vi "插入单条数据.vi"(8 "错误输入（无错误）":errorcluster, 10 "table输入":string(combo), 11 "插入数据":string[](array[string])) -> (0 "错误输出":errorcluster, 3 "远程数据":string[][](table))   [LabVIEW 2016]
uses:
  <vilib>/Utility/sysdir.llb/System Directory Type.ctl
  <vilib>/addons/database/Connection.llb/DB Tools Open Connec (String).vi
  <vilib>/addons/database/Connection.llb/Conn Execute.vi
  <vilib>/addons/database/Recordset.llb/Rec Destroy - Connection.vi
  <vilib>/addons/database/_DB Variant To Data/Database Variant To Data.xnode
  <vilib>/addons/database/NI_Database_API.lvlib
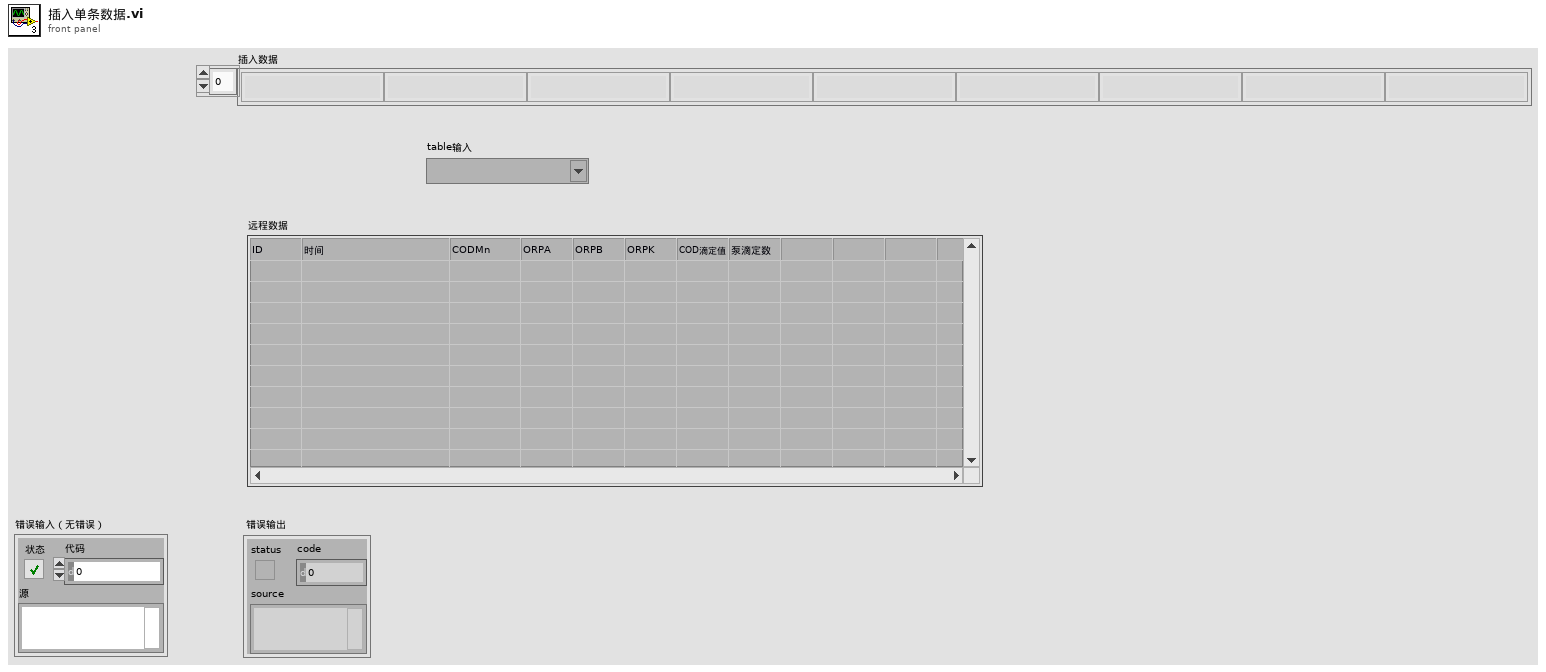
[diagram p1: front panel]
types:
  T1 = typedef "System Directory Type.ctl" = i32
  T2 = typedef "NI_Database_API.lvlib/Conn ObjectReference.ctl" = refnum<k1>
  T3 = typedef "NI_Database_API.lvlib/Rec ObjectReference.ctl" = refnum<k1>
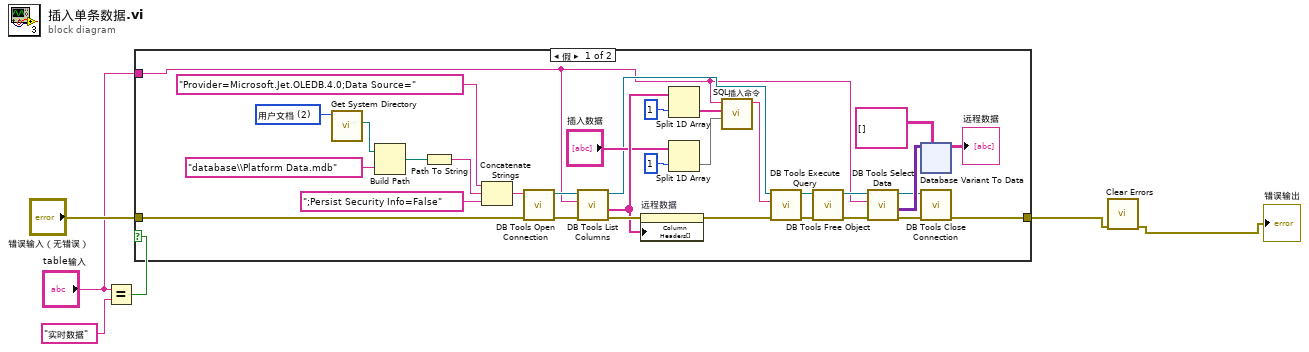
[diagram p0: block diagram]
diagram:
  n1 = Equal?(x="table输入", y="实时数据") -> (x = y?=w3:bool)
  n2 = case shown="假" w3 {
    tunnel: [w38 w83] -> w2
    tunnel: "错误输入（无错误）" -> [w20 w83]
    tunnel: "table输入" -> [w7 _]
    frame False {
      w21 = T1 2 items=["用户目录"=0, "用户桌面"=1, "用户文档"=2, "用户应用程序数据"=3, "用户设置"=4, "用户临时目录"=5, "公共文档"=6, "公共应用程序数据"=7, "公共设置"=8, "公共缓存"=13, "系统核心库"=9, "系统安装库"=10, "应用程序文件"=11, "启动盘根目录"=12] ("system directory type")
      n3 = call <vilib>:"Get System Directory.vi"("system directory type"=w21) -> ("system directory"=w23:path)  [unwired: 10 in]
      n4 = Build Path(base path=w23, name or relative path="database\\Platform Data.mdb" ("condition")) -> (appended path=w24:path)
      n5 = Path To String(path=w24) -> (string=w25:string)
      n6 = Concatenate Strings("Provider=Microsoft.Jet.OLEDB.4.0;Data Source=" ("condition"), w25, ";Persist Security Info=False" ("condition")) -> (w27:string)
      n7 = call-poly <vilib>:"DB Tools Open Connection.vi"("error in (no error)"=w20, "connection information"=w27) -> ("error out"=w36:errorcluster, "connection reference"=w35:T2)  [unwired: 6 in]
      n8 = call <vilib>:"DB Tools List Columns.vi"("error in (no error)"=w36, "table"=w7, "connection reference"=w35) -> ("error out"=w19:errorcluster, "columns"=w18:string[], "connection reference out"=w15:T2)  [unwired: 1 in, 1 out]
      n9 = property on="远程数据" class="Tbl (严格)"(error in=w19, "Column Headers[]"=w18) -> (error out=w14:errorcluster)  [unwired: 1 in, 1 out]
      n10 = Split 1D Array(array=w18, index=1 ("索引")) -> (second subarray=w9:string[])  [unwired: 1 out]
      n11 = Split 1D Array(array="插入数据", index=1 ("索引")) -> (second subarray=w8:string[])  [unwired: 1 out]
      n12 = call "SQL插入命令.vi"("插入数值"=w8, "段名"=w9, "table"=w7) -> ("SQL插入命令"=w16:string)  [unwired: 8 in]
      n13 = call-poly <vilib>:"DB Tools Execute Query.vi"("error in (no error)"=w14, "SQL query"=w16, "connection reference"=w15) -> ("error out"=w12:errorcluster, "recordset reference"=w13:T3)  [unwired: 5 in]
      n14 = call-poly <vilib>:"DB Tools Free Object.vi"("error in (no error)"=w12, "recordset reference"=w13) -> ("error out"=w10:errorcluster, "connection reference"=w11:T2)  [unwired: 8 in]
      n15 = call <vilib>:"DB Tools Select Data.vi"("error in (no error)"=w10, "table"=w7, "connection reference"=w11) -> ("error out"=w31:errorcluster, "data"=w33:variant[][], "connection reference out"=w32:T2)  [unwired: 3 in]
      n16 = xnode "Database Variant To Data"("database variant"=w33, "type"=string[][] []) -> ("data"=→"远程数据":string[][])  [unwired: 1 in, 1 out]
      n17 = call <vilib>:"DB Tools Close Connection.vi"("error in (no error)"=w31, "connection reference"=w32) -> ("error out"=w38:errorcluster)  [unwired: 5 in]
    }
    frame True {
    }
  }
  n18 = call <vilib>:"Clear Errors.vi"("error in (no error)"=w2) -> ("error out"=→"错误输出":errorcluster)  [unwired: 5 in, 1 out]
